vi "New UniqueObject.vi"(11 "UniqueName in":refnum<class "UniqueName.lvclass">) -> (3 "UniqueName out":refnum<class "UniqueName.lvclass">)   [LabVIEW 2013, in "UniqueName.lvlib" / "UniqueName.lvclass"]
uses:
  UniqueName.lvclass
  RandomStringGenerator/RandomStringGenerator.lvclass
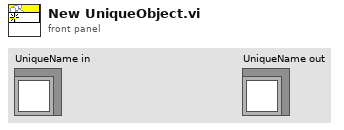
[diagram p1: front panel]
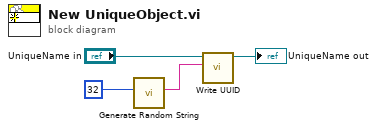
[diagram p0: block diagram]
diagram:
  n1 = call "Generate Random String.vi"("String Length (32)"=u32 32) -> ("Random String"=w2:string)  [unwired: 10 in]
  n2 = call "Write UUID.vi"("UUID"=w2, "UniqueName in"="UniqueName in") -> ("UniqueName out"=→"UniqueName out":refnum<class "UniqueName.lvclass">)  [unwired: 9 in]
